vi "Test_ReadItemAsVariant_Found_VariantValueOut.vi"(8 "error in (no error)":errorcluster, 11 "TestCase in":refnum<class "TestComposedLookupTable.lvclass">) -> (0 "error out":errorcluster, 3 "TestCase out":refnum<class "TestComposedLookupTable.lvclass">)   [LabVIEW 2017, in "TestComposedLookupTable.lvclass"]
uses:
  TestComposedLookupTable.lvclass
  Source/LookupTable/LookupTable.lvclass/LookupTable.ctl
  7b6ce473-d916-44cf-be00-7f0bb16d5bdf.vi
  01d6e16f-4164-4d05-a2e0-2f61dda92b48.vi
  Source/LookupTable/Read Table Reference.vi
  7b6ce473-d916-44cf-be00-7f0bb16d5bdf.vi/6b4e804c-7a9d-4c29-8e4f-427f14223bc0.vi
  01d6e16f-4164-4d05-a2e0-2f61dda92b48.vi/51725428-e383-498f-a867-24b3692aa066.vi
  Source/LookupTable/LookupTable.lvclass
panel:
  out "Value (as variant)":variant
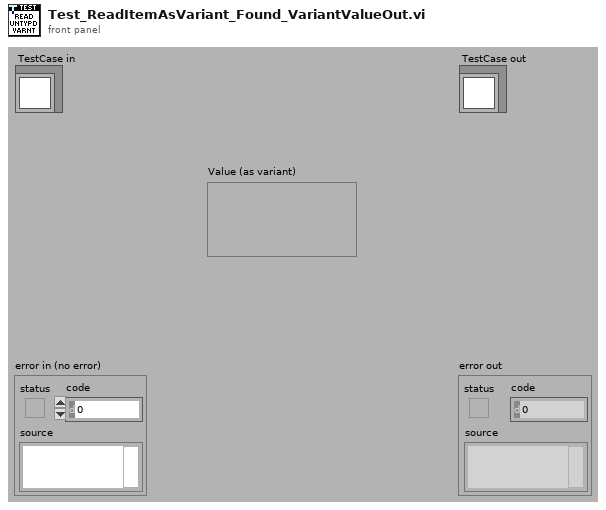
[diagram p1: front panel]
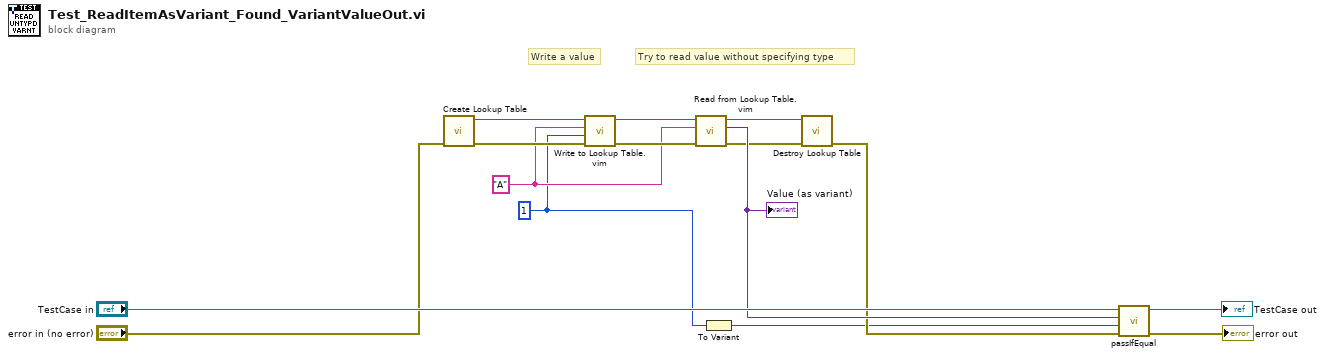
[diagram p0: block diagram]
diagram:
  w2 = 1
  w8 = "A" ("Item Name")
  # "Try to read value without specifying type"
  # "Write a value"
  n1 = call "Create Lookup Table.vi"("error in (no error)"="error in (no error)") -> ("error out"=w15:errorcluster, "LookupTable Reference"=w7:refnum<data-value>)  [unwired: 9 in]
  n2 = call "Write to Lookup Table.vim"("error in (no error)"=w15, "Item"=w2, "Item Name"=w8, "LookupTable Reference"=w7) -> ("error out"=w14:errorcluster, "LookupTable Reference Out"=w9:refnum<data-value>)  [unwired: 5 in, 1 out]
  n3 = call "Read from Lookup Table.vim"("error in (no error)"=w14, "Item Name"=w8, "LookupTable Reference"=w9) -> ("error out"=w4:errorcluster, "Value"=w10:variant, "LookupTable Reference Out"=w5:refnum<data-value>)  [unwired: 5 in, 1 out]
  "Value (as variant)" <- w10
  n4 = To Variant(anything=w2) -> (Variant=w1:variant)
  n5 = call "Destroy Lookup Table.vi"("error in (no error)"=w4, "LookupTable Reference"=w5) -> ("error out"=w3:errorcluster)  [unwired: 9 in]
  n6 = call-dynamic "passIfEqual.vi"("error in (no error)"=w3, "y"=w1, "x"=w10, "TestCase in"="TestCase in") -> ("error out"=→"error out":errorcluster, "TestCase out"=→"TestCase out":refnum<class "TestComposedLookupTable.lvclass">)  [unwired: 6 in]
